vi "LEBITplc.constructor.vi"(0 "name":string, 2 "data in":string, 5 "error in(no error)":errorcluster) -> (14 "i ref out":refnum<vi>, 16 "data out":string, 19 "error out":errorcluster)   [LabVIEW 2014, in "LEBITplc.lvlib"]
doc: "This is the constructor of a class.\n\nLicense Agreement for this software:\n\nCopyright (C)\nGesellschaft für Schwerionenforschung, GSI\nPlanckstr. 1\n64291 Darmstadt\nGermany\n\nContact: D.Beck@gsi.de \n\nThis program is free software; you can redistribute it and/or modify it under the terms of the \nGNU General Public License as published by the Free Software Foundation; either version 2 of \nthe license, or (at your option) any later version.\n\nThis program is distributed in the hope that it will be useful, but WITHOUT ANY WARRANTY; \nwithout even the implied warranty of MERCHANTABILITY or FITNESS FOR A PARTICULAR PURPOSE. See the GNU General License for more details (http://www.gnu.org).\n\nGesellschaft für Schwerionenforschung, GSI\nPlanckstr. 1, 64291 Darmstadt, Germany\nFor all questions and ideas contact: M.Richter@gsi.de, H.Brand@gsi.de or D.Beck@gsi.de.\nLast update: 16-JUN-2004"
uses:
  LEBITplc.lvlib
  CS_Core/BaseProcess/BaseProcess.lvlib
  CS_Core/CSSystem/CSSystemLib/CSSystemLib.lvlib
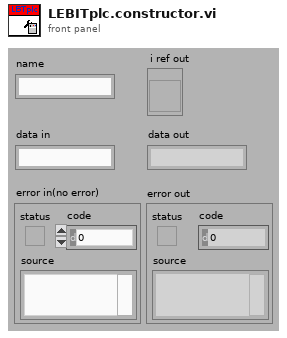
[diagram p1: front panel]
types:
  T1 = enum16{"SetAttribute", "GetAttribute", "CreateAttribute", "DestroyAttribute", "DestroyAllAtributes"}
  T2 = typedef "BaseProcess.lvlib/BaseProcess.i attribute.ctl" = cluster{"EventStatus":string, "EventError":i32, "PresetEvtWatchD":i32, "PresetPdcWatchD":i32, "EventTimeout":i32, "PeriodicInterval":i32, "Interface":string[], "Address":string[], "Special":string[], "PeriodicError":i32, "PeriodicStatus":string, "SuperProc":string, "Descriptors":T3[], "CaseRef":refnum<vi>, "PdcRef":refnum<vi>, "Thread Ref":refnum<vi>, "eventErrorID":i32, "eventStatusID":i32, "periodicErrorID":i32, "periodicStatusID":i32, "pdcCtrID":i32}
  T3 = typedef "BaseProcess.lvlib/BaseProcess.descriptor definition.ctl" = cluster{"selector":string, "descriptor":T4}
  T4 = typedef "BaseProcess.lvlib/BaseProcess.descriptor string definition.ctl" = string
  T5 = typedef "LEBITplc.lvlib/LEBITplc.i attribute.ctl" = cluster{"LLFLocation":string, "SetFileLocation":string, "nickNames":string[], "setValuePLCServiceID":i32[], "GUIServiceID":i32[], "monValuePLC":string[], "SetValueServiceID":i32[], "MonValueServiceID":i32[], "SetValue":dbl[][], "SetValueMin":dbl[], "SetValueMax":dbl[], "SetValueInfoServiceID":i32[], "GUINames":string[], "ListOfBases":string[], "Scale":dbl[], "Offset":dbl[], "setValuePLC":string[], "BaseName":string[], "ScaleServiceID":i32[], "OffsetServiceID":i32[], "AllPLCValues":string[], "CondSpecialArray":string[][], "CondSpecialIndex":i32[], "CondSpecialMonValue":dbl[], "RecentlyChanged":i32[], "SetFileLocationID":i32, "Dependent-Monitors":string[][], "LastLoadedFiles":string[], "IonGuideCalibLocation":string, "Monitor Dependent":string[], "Special":string[], "PLC?":bool[], "Start Date":string, "ListOfBasesServiceID":i32, "SETRA VISA resource":refnum<visa-resource-name>}
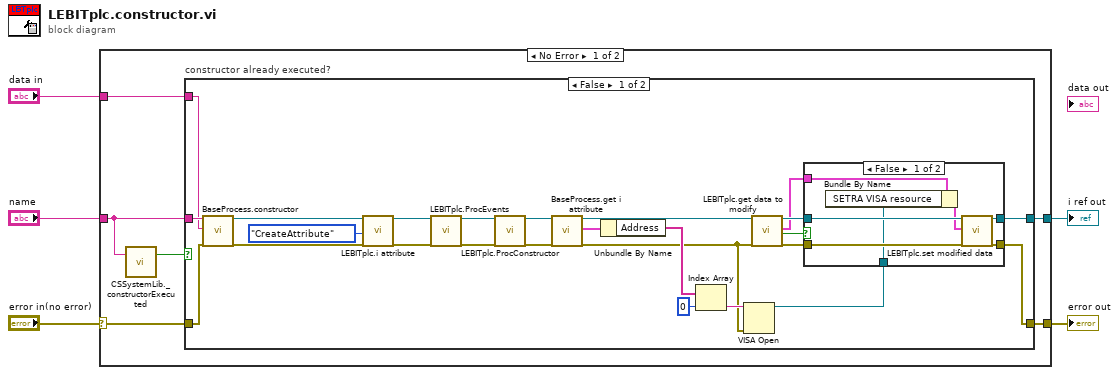
[diagram p0: block diagram]
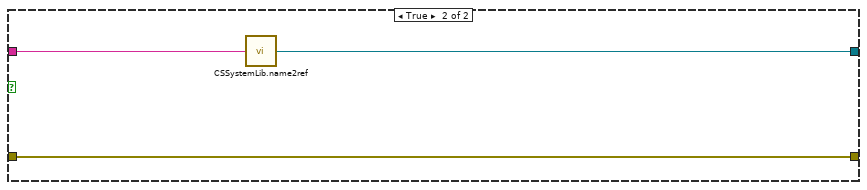
[diagram p3: hidden frame]
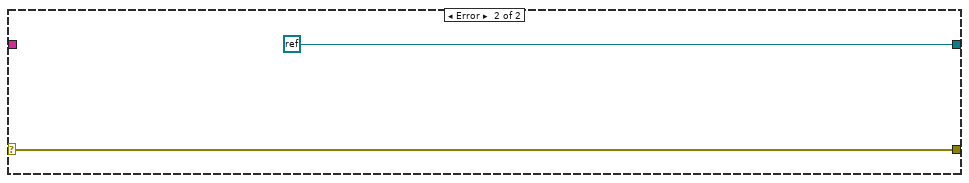
[diagram p4: hidden frame]
diagram:
  n1 = case shown="No Error" "error in(no error)" {
    selector: "error in(no error)" -> [w9 w49]
    tunnel: "name" -> [w8 _]
    tunnel: [w11 refnum<k0> refnum] -> w4
    tunnel: [w10 w49] -> w3
    tunnel: "data in" -> [w6 _]
    frame No Error {
      n2 = call "CSSystemLib._constructorExecuted.vi"("name"=w8) -> ("constructor executed?"=w7:bool)  [unwired: 18 in]
      n3 = case "constructor already executed?" shown="False" w7 {
        tunnel: [w15 w47] -> w11
        tunnel: [w14 w46] -> w10
        tunnel: w9 -> [w32 w46]
        tunnel: w8 -> [w31 w48]
        tunnel: w6 -> [w30 _]
        frame False {
          n4 = call "BaseProcess.constructor.vi"("name"=w31, "data in"=w30, "error in (no error)"=w32) -> ("i ref out"=w36:refnum<vi>, "error out"=w35:errorcluster)  [unwired: 14 in, 1 out]
          n5 = call "LEBITplc.i attribute.vi"("VI Refnum"=w36, "Action"=T1."CreateAttribute", "error in (no error)"=w35) -> ("VI Refnum out"=w34:refnum<vi>, "error out"=w33:errorcluster)  [unwired: 14 in, 1 out]
          n6 = call "LEBITplc.ProcEvents.vi"("i ref in"=w34, "error in"=w33) -> ("i ref out"=w27:refnum<vi>, "error out"=w28:errorcluster)  [unwired: 16 in]
          n7 = call "LEBITplc.ProcConstructor.vi"("i ref in"=w27, "error in(no error)"=w28) -> ("i ref out"=w21:refnum<vi>, "error out"=w22:errorcluster)  [unwired: 16 in]
          n8 = call "BaseProcess.get i attribute.vi"("i ref in"=w21, "error in (no error)"=w22) -> ("i ref out"=w20:refnum<vi>, "i attribute"=w26:T2, "error out"=w19:errorcluster)  [unwired: 15 in]
          n9 = Unbundle By Name(w26) -> ("Address"=w25:string[])
          n10 = Index Array(array=w25, index=0) -> (element=w23:string)
          n11 = VISA Open(error in (no error)=w19, VISA resource name=w23) -> (VISA resource name=w12:refnum<visa-resource-name>)  [unwired: 3 in, 1 out]
          n12 = call "LEBITplc.get data to modify.vi"("i ref in"=w20, "error in (no error)"=w19) -> ("i ref out"=w16:refnum<vi>, "i attribute"=w13:T5, "timed out"=w18:bool, "error out"=w17:errorcluster)  [unwired: 14 in]
          n13 = case shown="False" w18 {
            tunnel: w17 -> [w43 w44]
            tunnel: w16 -> [w42 w45]
            tunnel: [w41 w45] -> w15
            tunnel: [w40 w44] -> w14
            tunnel: w13 -> [w39 _]
            tunnel: w12 -> [w37 _]
            frame False {
              n14 = Bundle By Name(cluster=w39, "SETRA VISA resource"=w37) -> (w38:T5)
              n15 = call "LEBITplc.set modified data.vi"("i ref in"=w42, "i attribute"=w38, "error in (no error)"=w43) -> ("i ref out"=w41:refnum<vi>, "error out"=w40:errorcluster)  [unwired: 15 in]
            }
            frame True {
            }
          }
        }
        frame True {
          n16 = call "CSSystemLib.name2ref.vi"("name"=w48) -> ("obj refnum"=w47:refnum<vi>)
        }
      }
    }
    frame Error {
    }
  }
  "i ref out" <- w4
  "error out" <- w3
